vi "Global Memory.vi"() -> ()   [LabVIEW 2026, in "TALOS.lvlib"]
uses:
  TALOS.lvlib
  Classes/Error Filter/Error Filter.lvclass
  Interfaces/FPGA Interface/FPGA Interface.lvclass
panel:
  out "Suppress error window":bool=TRUE
  in  "FPGA Interface":refnum<class "FPGA Interface.lvclass">
  out "DAQ Sender Name":string
  out "Crit PCs List":string[](array[string])
  out "FPGA List":string[](array[string])
  out "FPGA IPs Map":map{string, string}(c390)
  out "DAQ DLL Path":path
  out "Run Number":i32
  out "DAQ Address":cluster{"Port":u16, "Path":string}
  out "Error Filter DVR":refnum<data-value>
  out "Circus Error Criticality":u8[](array[numeric])
  out "TALOS Root Path":path
  out "Circus Root Path":path
  out "Is in Packed Library?":bool
  out "Circus Error Messages":string[](array[string])
  out "Circus Error Codes":i32[](array[numeric])
  out "PC Name":string
  out "PCs IPs Map":map{string, string}(c390)
  out "Circus Config Param Map":map{string, string}(c390)
  out "TALOS Config Param Map":map{string, string}(c390)
  out "PCs List":string[](array[string])
  # "They should become a unique object"
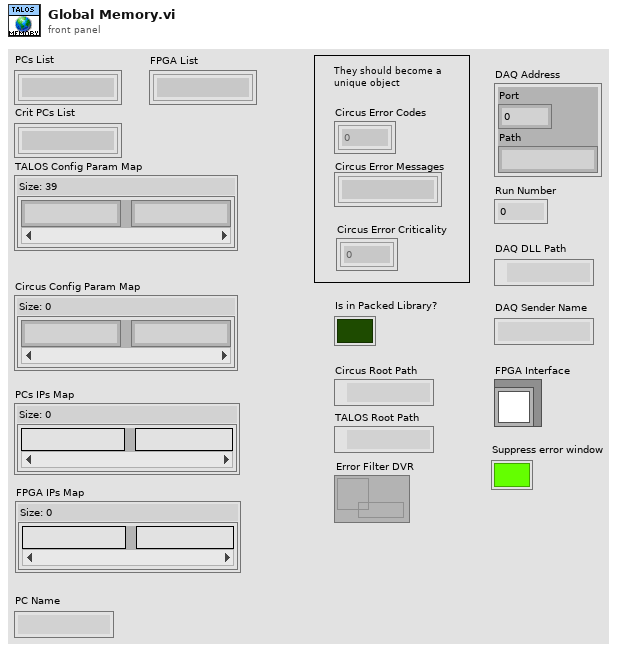
[diagram p1: front panel]
diagram:
